vi "Configure Bandwidth Search.vi"(5 "Marker (1)":i32=1, 6 "Bandwidth Definition Value (-3.0)":dbl=-3.0 format="%.2f", 7 "Channel (1)":i32=1, 8 "error in (no error)":errorcluster, 10 "Result Display State (F: Disable)":bool, 11 "VISA resource name":refnum<visa-resource-name>) -> (0 "error out":errorcluster, 3 "VISA resource name out":refnum<visa-resource-name>)   [LabVIEW 2012, in "Tektronix TTR500 Series.lvlib"]
doc: "This VI configures bandwidth marker search."
uses:
  <instrlib>/Tektronix TTR500 Series/Tektronix TTR500 Series.lvlib
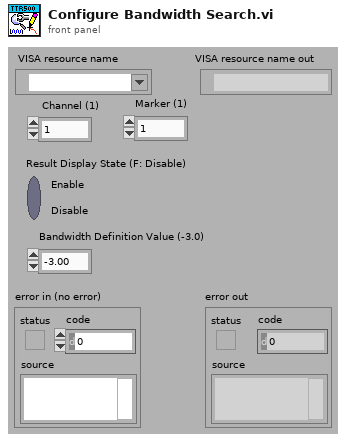
[diagram p1: front panel]
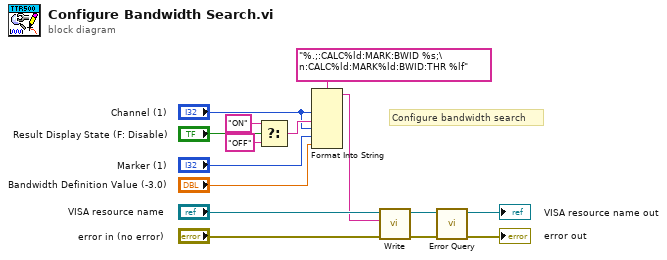
[diagram p0: block diagram]
diagram:
  # "Configure bandwidth search"
  n1 = Select(t="ON", s="Result Display State (F: Disable)", f="OFF") -> (s? t:f=w10:string)
  n2 = Format Into String(format string="%.;:CALC%ld:MARK:BWID %s;\n:CALC%ld:MARK%ld:BWID:THR %lf", "Channel (1)", w10, "Channel (1)", "Marker (1)", "Bandwidth Definition Value (-3.0)") -> (resulting string=w5:string)  [unwired: 2 in, 1 out]
  n3 = call <instrlib>:"Write.vi"("error in (no error)"="error in (no error)", "String ()"=w5, "VISA resource name"="VISA resource name") -> ("error out"=w3:errorcluster, "VISA resource name out"=w4:refnum<visa-resource-name>)  [unwired: 6 in, 1 out]
  n4 = call <instrlib>:"Error Query.vi"("error in (no error)"=w3, "VISA resource name"=w4) -> ("error out"=→"error out":errorcluster, "VISA resource name out"=→"VISA resource name out":refnum<visa-resource-name>)  [unwired: 6 in, 2 out]
